vi "Encoder Data.vi"() -> ()   [LabVIEW 2013]
panel:
  in  "Encoder 2 Data":cluster{dbl, "String":string}
  in  "Encoder 1 Data":cluster{dbl, "String":string}
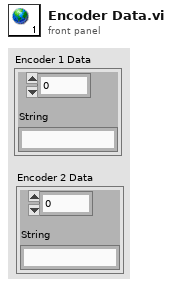
[diagram p1: front panel]
diagram:
